vi "Execute.vi"(8 "error in (no error)":errorcluster, 11 "Node in":refnum<class "Assign abs_Value.lvclass">) -> (0 "error out":errorcluster, 1 "Status":T1, 3 "Node out":refnum<class "Assign abs_Value.lvclass">)   [LabVIEW 2021, in "BT.lvlib" / "Assign abs_Value.lvclass"]
uses:
  Assign abs_Value.lvclass
  abs_Node/Status.ctl
  Assign abs_Value.lvclass/Assign abs_Value.ctl
  <vilib>/TSA/Abstract Data Classes/Abs_Types/Value/Abs_Value.lvclass
  abs_Node/bt_Node.lvclass
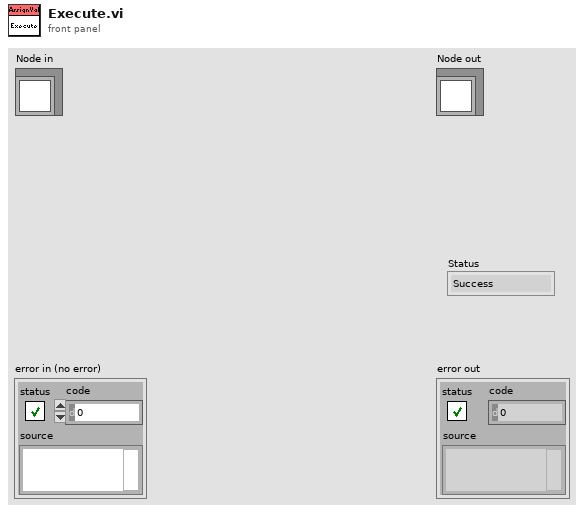
[diagram p1: front panel]
types:
  T1 = typedef "BT.lvlib/bt_Node.lvclass/Status.ctl" = enum16{"Success", "Failure", "Running"}
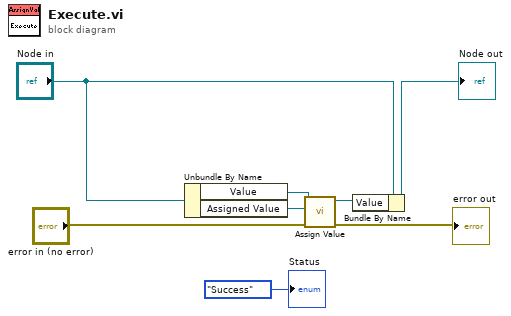
[diagram p0: block diagram]
diagram:
  n1 = Unbundle By Name("Node in") -> ("Value"=w4:refnum<class "Abs_Value.lvclass">, "Assigned Value"=w3:refnum<class "Abs_Value.lvclass">)
  n2 = call-dynamic "Assign Value.vi"("error in (no error)"="error in (no error)", "Assigned Value"=w3, "Abs_Value in"=w4) -> ("error out"=→"error out":errorcluster, "Abs_Value out"=w1:refnum<class "Abs_Value.lvclass">)  [unwired: 7 in]
  n3 = Bundle By Name(cluster="Node in", "Value"=w1) -> (→"Node out":refnum<class "Assign abs_Value.lvclass">)
  "Status" <- Status."Success" ("Status")
